vi "Convert 16xIQpair to 16IQdata.vi"(10 "16xIQpair in":T1=[{"I"=0.0, "Q"=0.0}, {"I"=0.0, "Q"=0.0}, {"I"=0.0, "Q"=0.0}, {"I"=0.0, "Q"=0.0}, {"I"=0.0, "Q"=0.0}, {"I"=0.0, "Q"=0.0}, {"I"=0.0, "Q"=0.0}, {"I"=0.0, "Q"=0.0}, {"I"=0.0, "Q"=0.0}, {"I"=0.0, "Q"=0.0}, {"I"=0.0, "Q"=0.0}, {"I"=0.0, "Q"=0.0}, {"I"=0.0, "Q"=0.0}, {"I"=0.0, "Q"=0.0}, {"I"=0.0, "Q"=0.0}, {"I"=0.0, "Q"=0.0}]) -> (2 "16xIQdata out":T2)   [LabVIEW 2015, in "DDC_7976R_v1.lvlib"]
uses:
  DDC_7976R_v1.lvlib
  16xIQData.ctl
  <instrlib>/_niInstr/DSP/v1/Shared/Public/IQ Data.ctl
  16xIQData_without_overflow.ctl
  <instrlib>/_niInstr/DSP/v1/Shared/niInstr DSP v1 Shared.lvlib
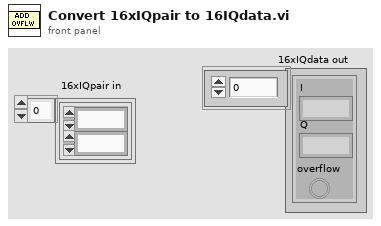
[diagram p1: front panel]
types:
  T1 = typedef "DDC_7976R_v1.lvlib/16xIQData_without_overflow.ctl" = cluster{"I":fxp<+/-,18,1>, "Q":fxp<+/-,18,1>}[]
  T2 = typedef "DDC_7976R_v1.lvlib/16xIQData.ctl" = T3[]
  T3 = typedef "niInstr DSP v1 Shared.lvlib/IQ Data.ctl" = cluster{"I":fxp<+/-,18,1>, "Q":fxp<+/-,18,1>, "overflow":bool}
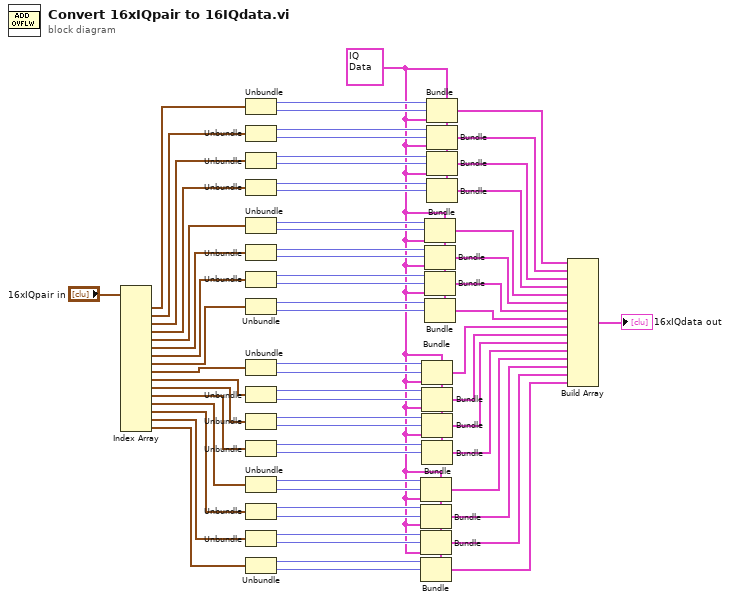
[diagram p0: block diagram]
diagram:
  w1 = T3 {"I"=0.0, "Q"=0.0, "overflow"=FALSE} ("data")
  n1 = Index Array(array="16xIQpair in") -> (element #1=w67:cluster{"I":fxp<+/-,18,1>, "Q":fxp<+/-,18,1>}, element #2=w66:cluster{"I":fxp<+/-,18,1>, "Q":fxp<+/-,18,1>}, element #3=w65:cluster{"I":fxp<+/-,18,1>, "Q":fxp<+/-,18,1>}, element #4=w64:cluster{"I":fxp<+/-,18,1>, "Q":fxp<+/-,18,1>}, element #5=w63:cluster{"I":fxp<+/-,18,1>, "Q":fxp<+/-,18,1>}, element #6=w62:cluster{"I":fxp<+/-,18,1>, "Q":fxp<+/-,18,1>}, element #7=w61:cluster{"I":fxp<+/-,18,1>, "Q":fxp<+/-,18,1>}, element #8=w60:cluster{"I":fxp<+/-,18,1>, "Q":fxp<+/-,18,1>}, element #9=w59:cluster{"I":fxp<+/-,18,1>, "Q":fxp<+/-,18,1>}, element #10=w58:cluster{"I":fxp<+/-,18,1>, "Q":fxp<+/-,18,1>}, element #11=w57:cluster{"I":fxp<+/-,18,1>, "Q":fxp<+/-,18,1>}, element #12=w56:cluster{"I":fxp<+/-,18,1>, "Q":fxp<+/-,18,1>}, element #13=w55:cluster{"I":fxp<+/-,18,1>, "Q":fxp<+/-,18,1>}, element #14=w54:cluster{"I":fxp<+/-,18,1>, "Q":fxp<+/-,18,1>}, element #15=w53:cluster{"I":fxp<+/-,18,1>, "Q":fxp<+/-,18,1>}, element #16=w52:cluster{"I":fxp<+/-,18,1>, "Q":fxp<+/-,18,1>})  [unwired: 16 in]
  n2 = Unbundle(w67) -> ("I"=w51:fxp<+/-,18,1>, "Q"=w50:fxp<+/-,18,1>)
  n3 = Unbundle(w66) -> ("I"=w49:fxp<+/-,18,1>, "Q"=w48:fxp<+/-,18,1>)
  n4 = Unbundle(w65) -> ("I"=w47:fxp<+/-,18,1>, "Q"=w46:fxp<+/-,18,1>)
  n5 = Unbundle(w64) -> ("I"=w45:fxp<+/-,18,1>, "Q"=w44:fxp<+/-,18,1>)
  n6 = Unbundle(w63) -> ("I"=w43:fxp<+/-,18,1>, "Q"=w42:fxp<+/-,18,1>)
  n7 = Unbundle(w62) -> ("I"=w41:fxp<+/-,18,1>, "Q"=w40:fxp<+/-,18,1>)
  n8 = Unbundle(w61) -> ("I"=w39:fxp<+/-,18,1>, "Q"=w38:fxp<+/-,18,1>)
  n9 = Unbundle(w60) -> ("I"=w37:fxp<+/-,18,1>, "Q"=w36:fxp<+/-,18,1>)
  n10 = Unbundle(w59) -> ("I"=w35:fxp<+/-,18,1>, "Q"=w34:fxp<+/-,18,1>)
  n11 = Unbundle(w58) -> ("I"=w33:fxp<+/-,18,1>, "Q"=w32:fxp<+/-,18,1>)
  n12 = Unbundle(w57) -> ("I"=w31:fxp<+/-,18,1>, "Q"=w30:fxp<+/-,18,1>)
  n13 = Unbundle(w56) -> ("I"=w29:fxp<+/-,18,1>, "Q"=w28:fxp<+/-,18,1>)
  n14 = Unbundle(w55) -> ("I"=w27:fxp<+/-,18,1>, "Q"=w26:fxp<+/-,18,1>)
  n15 = Unbundle(w54) -> ("I"=w25:fxp<+/-,18,1>, "Q"=w24:fxp<+/-,18,1>)
  n16 = Unbundle(w53) -> ("I"=w23:fxp<+/-,18,1>, "Q"=w22:fxp<+/-,18,1>)
  n17 = Unbundle(w52) -> ("I"=w21:fxp<+/-,18,1>, "Q"=w20:fxp<+/-,18,1>)
  n18 = Bundle(cluster=w1, "I"=w27, "Q"=w26) -> (w7:T3)  [unwired: 1 in]
  n19 = Bundle(cluster=w1, "I"=w25, "Q"=w24) -> (w6:T3)  [unwired: 1 in]
  n20 = Bundle(cluster=w1, "I"=w23, "Q"=w22) -> (w5:T3)  [unwired: 1 in]
  n21 = Bundle(cluster=w1, "I"=w21, "Q"=w20) -> (w4:T3)  [unwired: 1 in]
  n22 = Bundle(cluster=w1, "I"=w35, "Q"=w34) -> (w11:T3)  [unwired: 1 in]
  n23 = Bundle(cluster=w1, "I"=w33, "Q"=w32) -> (w10:T3)  [unwired: 1 in]
  n24 = Bundle(cluster=w1, "I"=w31, "Q"=w30) -> (w9:T3)  [unwired: 1 in]
  n25 = Bundle(cluster=w1, "I"=w29, "Q"=w28) -> (w8:T3)  [unwired: 1 in]
  n26 = Bundle(cluster=w1, "I"=w43, "Q"=w42) -> (w15:T3)  [unwired: 1 in]
  n27 = Bundle(cluster=w1, "I"=w41, "Q"=w40) -> (w14:T3)  [unwired: 1 in]
  n28 = Bundle(cluster=w1, "I"=w39, "Q"=w38) -> (w13:T3)  [unwired: 1 in]
  n29 = Bundle(cluster=w1, "I"=w37, "Q"=w36) -> (w12:T3)  [unwired: 1 in]
  n30 = Bundle(cluster=w1, "I"=w51, "Q"=w50) -> (w19:T3)  [unwired: 1 in]
  n31 = Bundle(cluster=w1, "I"=w49, "Q"=w48) -> (w18:T3)  [unwired: 1 in]
  n32 = Bundle(cluster=w1, "I"=w47, "Q"=w46) -> (w17:T3)  [unwired: 1 in]
  n33 = Bundle(cluster=w1, "I"=w45, "Q"=w44) -> (w16:T3)  [unwired: 1 in]
  n34 = Build Array(w19, w18, w17, w16, w15, w14, w13, w12, w11, w10, w9, w8, w7, w6, w5, w4) -> (→"16xIQdata out":T3[])
